vi "Insert Into Array.vi"(4 "error in (no error)":errorcluster, 5 "new element":refnum<class "Generic Plugin.lvclass">, 6 "index (end)":i32=-1, 7 "Controller Array in":refnum<class "Controller Array.lvclass">) -> (0 "error out":errorcluster, 2 "new element":refnum<class "Generic Plugin.lvclass">, 3 "Controller Array out":refnum<class "Controller Array.lvclass">)   [LabVIEW 2020, in "Controller Array.lvclass"]
doc: "Insert an element into the array at the specified index."
uses:
  Controller Array.lvclass
  Controller/Generic Plugin.lvclass
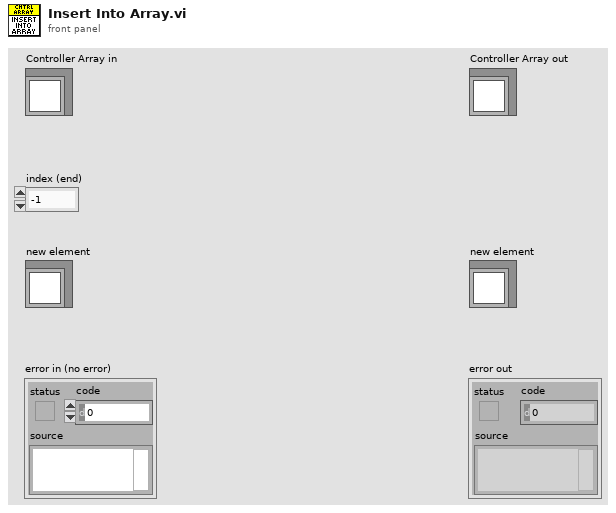
[diagram p1: front panel]
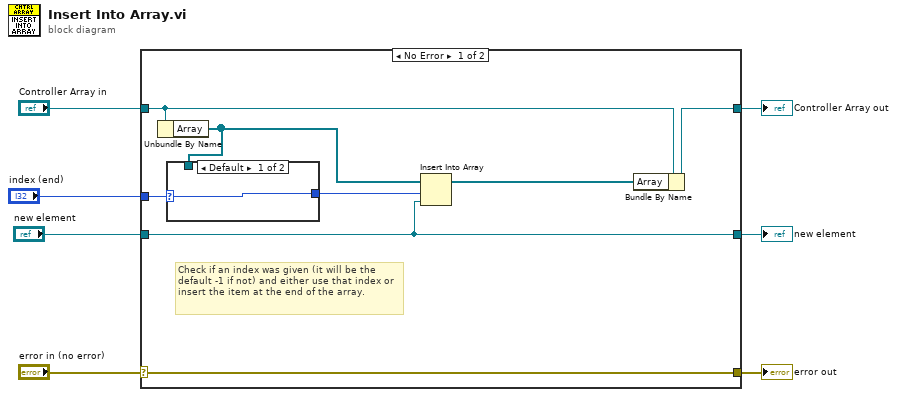
[diagram p0: block diagram]
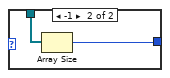
[diagram p2: hidden frame]
diagram:
  n1 = case shown="No Error" "error in (no error)" {
    selector: "error in (no error)" -> [w15 w21]
    tunnel: [w15 w21] -> w6
    tunnel: [w13 w20] -> w4
    tunnel: "Controller Array in" -> [w14 w20]
    tunnel: "index (end)" -> [w11 _]
    tunnel: "new element" -> [w8 w19]
    tunnel: [w8 w19] -> w1
    frame No Error {
      # "Check if an index was given (it will be the default -1 if not) and either use that index or insert the item at the end of the array."
      n2 = Unbundle By Name(w14) -> ("Array"=w10:refnum<class "Generic Plugin.lvclass">[])
      n3 = case shown="Default" w11 {
        selector: w11 -> [w16 _]
        tunnel: w10 -> [_ w18]
        tunnel: [w16 w17] -> w9
        frame Default {
        }
        frame -1 {
          n4 = Array Size(array=w18) -> (size(s)=w17:i32)
        }
      }
      n5 = Insert Into Array(array=w10, index=w9, new element=w8) -> (w12:refnum<class "Generic Plugin.lvclass">[])
      n6 = Bundle By Name(cluster=w14, "Array"=w12) -> (w13:refnum<class "Controller Array.lvclass">)
    }
    frame Error {
    }
  }
  "error out" <- w6
  "Controller Array out" <- w4
  "new element" <- w1
